vi "get runtime class name.vi"(8 "error in":errorcluster, 11 "configuration in":refnum<class "Template Action Cfg.lvclass">) -> (0 "error out":errorcluster, 2 "class name":string, 3 "configuration out":refnum<class "Template Action Cfg.lvclass">)   [LabVIEW 2014, in "Template Action Cfg.lvclass"]
doc: "Provides an interface for determining the runtime class associated with this configuration. This class name can then be used to dynamically load or locate the runtime class for initialization purposes."
uses:
  Template Action Cfg.lvclass
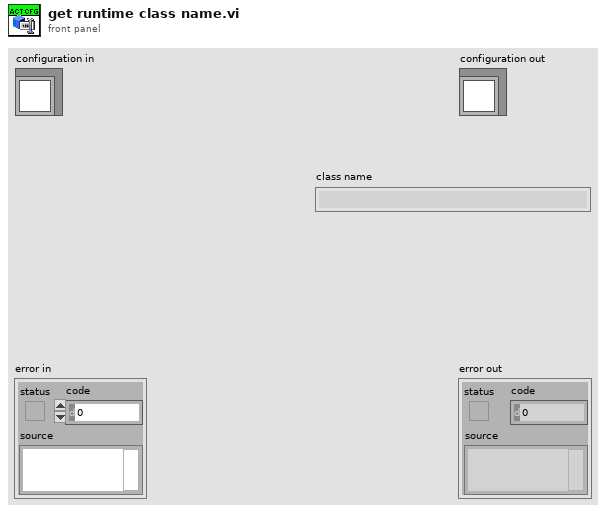
[diagram p1: front panel]
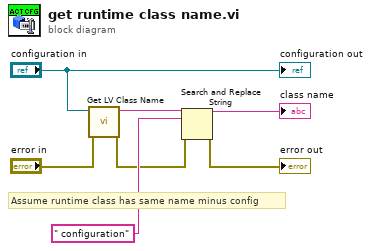
[diagram p0: block diagram]
diagram:
  # "Assume runtime class has same name minus config"
  n1 = call <vilib>:"Get LV Class Name.vi"("error in (no error)"="error in", "object"="configuration in") -> ("error out"=w2:errorcluster, "class name"=w5:string)  [unwired: 8 in]
  n2 = Search and Replace String(input string=w5, search string=" configuration", error in=w2) -> (result string=→"class name":string, error out=→"error out":errorcluster)  [unwired: 5 in, 2 out]
  "configuration out" <- "configuration in"
